vi "Print VI Panel or Documentation.vi"   [LabVIEW 2020, in "NI_ReportGenerationCore.lvlib"]
doc: "Prints a front panel or VI documentation or saves the front panel or VI documentation to a report."
uses:
  <vilib>/Utility/NIReport.llb/NI_ReportGenerationCore.lvlib
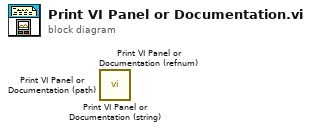
[diagram p0: block diagram]
diagram:
  n1 = call <vilib>:"Print VI Panel or Documentation (string).vi"() -> ()  [unwired: 10 in, 2 out]
  n2 = call <vilib>:"Print VI Panel or Documentation (refnum).vi"() -> ()  [unwired: 10 in, 2 out]
  n3 = call <vilib>:"Print VI Panel or Documentation (path).vi"() -> ()  [unwired: 10 in, 2 out]
